vi "Write configuration.vi"(8 "error in":errorcluster, 10 "configuration":refnum<class "NISE_CEF_serializable configuration.lvclass">, 11 "fixed channel editor in":refnum<class "fixed channel editor.lvclass">) -> (0 "error out":errorcluster, 3 "fixed channel editor out":refnum<class "fixed channel editor.lvclass">)   [LabVIEW 2013, in "fixed channel editor.lvclass"]
uses:
  fixed channel editor.lvclass
  <vilib>/NI/Configuration Framework/serializable configuration/NISE_CEF_serializable configuration.lvclass
  module/configuration/fixed channel configuration.lvclass
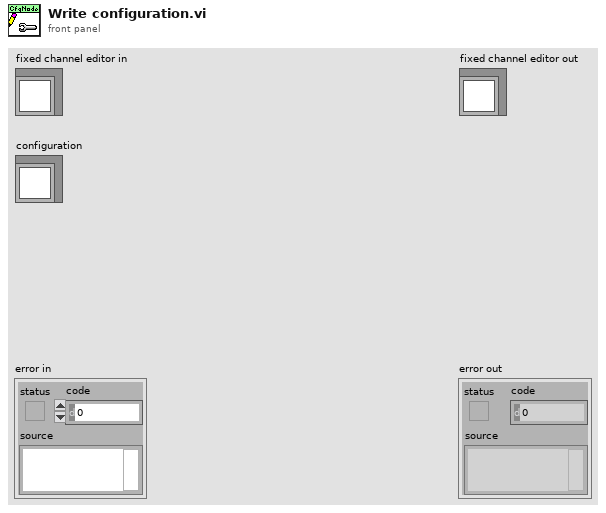
[diagram p1: front panel]
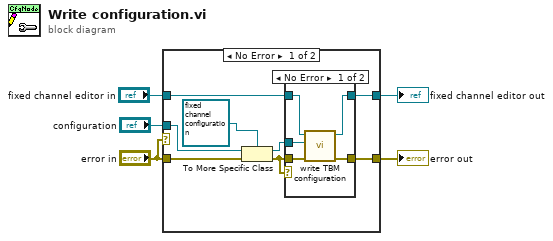
[diagram p0: block diagram]
diagram:
  n1 = case shown="No Error" "error in" {
    tunnel: [w13 w22] -> w5
    tunnel: "fixed channel editor in" -> [w12 w22]
    tunnel: "error in" -> [w11 w21]
    tunnel: [w10 w21] -> w3
    tunnel: "configuration" -> [w9 _]
    frame No Error {
      n2 = To More Specific Class(target class=refnum<class "fixed channel configuration.lvclass"> refnum ("fixed channel configuration"), reference=w9, error in=w11) -> (specific class reference=w7:refnum<class "fixed channel configuration.lvclass">, error out=w6:errorcluster)
      n3 = case shown="No Error" w6 {
        tunnel: [w18 w19] -> w13
        tunnel: w12 -> [w17 w19]
        tunnel: [w16 w20] -> w10
        tunnel: w6 -> [w15 w20]
        tunnel: w7 -> [w14 _]
        frame No Error {
          n4 = call-dynamic "write TBM configuration.vi"("error in"=w15, "configuration"=w14, "fixed module parent implementation editor node in"=w17) -> ("error out"=w16:errorcluster, "fixed module parent implementation editor node out"=w18:refnum<class "fixed channel editor.lvclass">)  [unwired: 7 in]
        }
        frame Error {
        }
      }
    }
    frame Error {
    }
  }
  "error out" <- w3
  "fixed channel editor out" <- w5
